vi "Load Save Config.vi"(8 "error in (no error)":errorcluster, 10 "OM  Location":T1, 11 "Actions":T2=enum."Load") -> (0 "error out":errorcluster)   [LabVIEW 2009]
uses:
  Data Access Objects/Metadata/Persistant DAO Actions.ctl
  Data Access Objects/Metadata/LBCB Location.ctl
  ConfigPathActions.ctl
  Data Access Objects/Metadata/LBCB Number.ctl
  <vilib>/Utility/config.llb/NI_LVConfig.lvlib
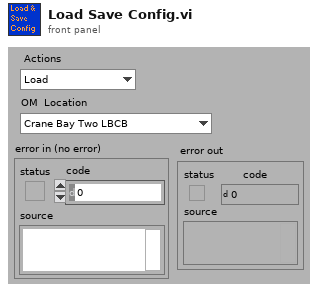
[diagram p1: front panel]
types:
  T1 = typedef "LBCB Location.ctl" = enum16{"Crane Bay Two LBCB", "Crane Bay One LBCB", "5th Scale Two LBCB", "5th Scale One LBCB", "Portable LBCB"}
  T2 = typedef "Persistant DAO Actions.ctl" = enum16{"Init", "Get", "Set", "Load", "Save"}
  T3 = typedef "ConfigPathActions.ctl" = enum16{"Init", "Application", "MixedMode", "ControlLoop", "Calibration", "System", "Change Location"}
  T4 = typedef "LBCB Number.ctl" = enum16{"LBCB1", "LBCB2"}
  T5 = typedef "NI_LVConfig.lvlib/Config Data RefNum.ctl" = refnum<k1>
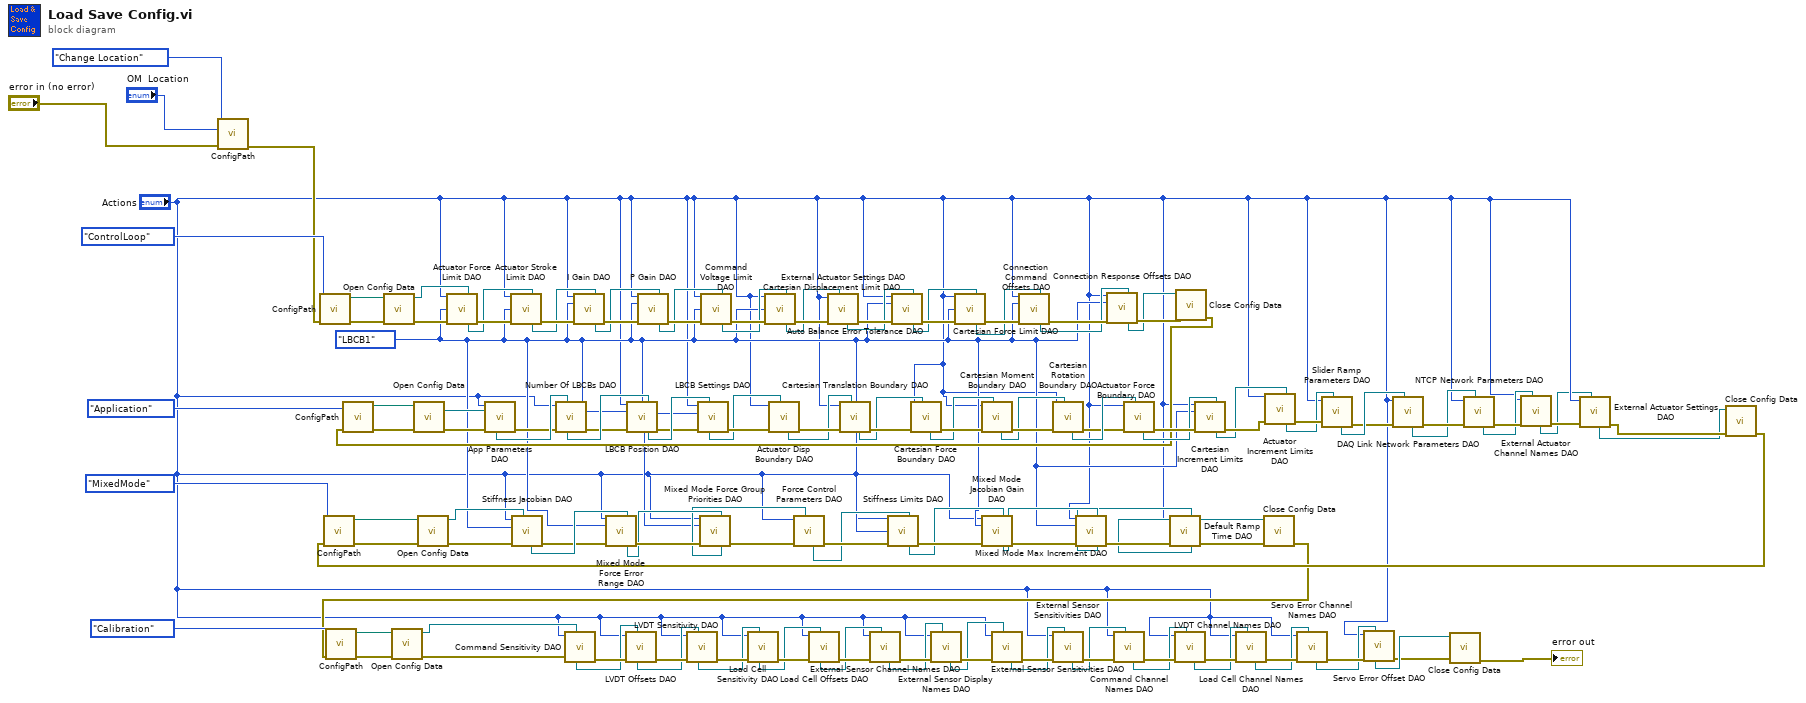
[diagram p0: block diagram]
diagram:
  w12 = LBCB_Number."LBCB1" ("LBCB Number")
  n1 = call "ConfigPath.vi"("error in (no error)"="error in (no error)", "OM  Location"="OM  Location", "Config Path Actions"=ConfigPathActions."Change Location") -> ("error out"=w89:errorcluster)  [unwired: 8 out]
  n2 = call "ConfigPath.vi"("error in (no error)"=w89, "Config Path Actions"=ConfigPathActions."ControlLoop") -> ("error out"=w130:errorcluster, "Path"=w129:path)  [unwired: 1 in, 7 out]
  n3 = call <vilib>:"Open Config Data.vi"("error in (no error)"=w130, "configuration file path"=w129) -> ("error out"=w127:errorcluster, "refnum"=w126:T5)  [unwired: 7 in, 1 out]
  n4 = call "Actuator Force Limit DAO.vi"("Actuator Force Limit Actions"="Actions", "Config Ref Number"=w126, "ID"=w12, "error in (no error)"=w127) -> ("Config Ref Number out"=w117:T5, "error out"=w125:errorcluster)  [unwired: 1 in, 9 out]
  n5 = call "Actuator Stroke Limit DAO.vi"("Actuator Stroke Limit Actions"="Actions", "Config Ref Number"=w117, "ID"=w12, "error in (no error)"=w125) -> ("Config Ref Number out"=w116:T5, "error out"=w124:errorcluster)  [unwired: 1 in, 9 out]
  n6 = call "I Gain DAO.vi"("I Gain Actions"="Actions", "Config Ref Number"=w116, "LBCB Number"=w12, "error in (no error)"=w124) -> ("Config Ref Number out"=w115:T5, "error out"=w123:errorcluster)  [unwired: 1 in, 9 out]
  n7 = call "P Gain DAO.vi"("P Gain Actions"="Actions", "Config Ref Number"=w115, "LBCB Number"=w12, "error in (no error)"=w123) -> ("Config Ref Number out"=w114:T5, "error out"=w122:errorcluster)  [unwired: 1 in, 9 out]
  n8 = call "Command Voltage Limit DAO.vi"("Actuator Stroke Limit Actions"="Actions", "Config Ref Number"=w114, "ID"=w12, "error in (no error)"=w122) -> ("Config Ref Number out"=w113:T5, "error out"=w121:errorcluster)  [unwired: 1 in, 9 out]
  n9 = call "Cartesian Displacement Limit DAO.vi"("Cartesian Displacement Limit Actions"="Actions", "Config Ref Number"=w113, "ID"=w12, "error in (no error)"=w121) -> ("Config Ref Number out"=w112:T5, "error out"=w120:errorcluster)  [unwired: 1 in, 9 out]
  n10 = call "External Actuator Settings DAO.vi"("refnum"=w112, "error in (no error)"=w120, "Persistent DAO Actions"="Actions") -> ("error out"=w119:errorcluster, "refnum out"=w111:T5)  [unwired: 2 in, 5 out]
  n11 = call "Auto Balance Error Tolerance DAO.vi"("Auto Balance Increment Actions"="Actions", "Config Ref"=w111, "LBCB Number"=w12, "error in (no error)"=w119) -> ("Config Ref  out"=w110:T5, "error out"=w118:errorcluster)  [unwired: 1 in, 9 out]
  n12 = call "Cartesian Force Limit DAO.vi"("Cartesian Force Limit Actions"="Actions", "Config Ref Number"=w110, "ID"=w12, "error in (no error)"=w118) -> ("Config Ref Number out"=w15:T5, "error out"=w19:errorcluster)  [unwired: 1 in, 9 out]
  n13 = call "Connection Command Offsets DAO.vi"("Actions"="Actions", "Config Ref Number"=w15, "LBCB Number"=w12, "error in (no error)"=w19) -> ("Config Ref Number out"=w14:T5, "error out"=w18:errorcluster)  [unwired: 9 in, 1 out]
  n14 = call "Connection Response Offsets DAO.vi"("Actions"="Actions", "Config Ref Number"=w14, "LBCB Number"=w12, "error in (no error)"=w18) -> ("Config Ref Number out"=w13:T5, "error out"=w17:errorcluster)  [unwired: 9 in, 1 out]
  n15 = call <vilib>:"Close Config Data.vi"("error in (no error)"=w17, "refnum"=w13) -> ("error out"=w16:errorcluster)  [unwired: 1 in, 8 out]
  n16 = call "ConfigPath.vi"("error in (no error)"=w16, "Config Path Actions"=ConfigPathActions."Application") -> ("error out"=w109:errorcluster, "Path"=w108:path)  [unwired: 1 in, 7 out]
  n17 = call <vilib>:"Open Config Data.vi"("error in (no error)"=w109, "configuration file path"=w108) -> ("error out"=w106:errorcluster, "refnum"=w105:T5)  [unwired: 7 in, 1 out]
  n18 = call "App Parameters DAO.vi"("config ref in"=w105, "error in (no error)"=w106, "Actions"="Actions") -> ("error out"=w87:errorcluster, "config ref out"=w88:T5)  [unwired: 1 in, 6 out]
  n19 = call "Number Of LBCBs DAO.vi"("Config ref in"=w88, "error in (no error)"=w87, "Actions"="Actions") -> ("error out"=w92:errorcluster, "Config ref out"=w94:T5)  [unwired: 2 in, 5 out]
  n20 = call "LBCB Position DAO.vi"("LBCB Settings Actions"="Actions", "Config Ref Number"=w94, "LBCB Number"=w12, "error in (no error)"=w92) -> ("Config Ref Number out"=w93:T5, "error out"=w91:errorcluster)  [unwired: 1 in, 9 out]
  n21 = call "LBCB Settings DAO.vi"("Config ref in"=w93, "error in (no error)"=w91, "LBCB Number"=w12, "Actions"="Actions") -> ("error out"=w81:errorcluster, "Config ref out"=w80:T5)  [unwired: 1 in, 5 out]
  n22 = call "Actuator Disp Boundary DAO.vi"("refnum in"=w80, "error in (no error)"=w81, "Actions"="Actions") -> ("error out"=w85:errorcluster, "refnum out"=w79:T5)  [unwired: 1 in, 6 out]
  n23 = call "Cartesian Translation Boundary DAO.vi"("refnum in"=w79, "error in (no error)"=w85, "Actions"="Actions") -> ("error out"=w84:errorcluster, "refnum out"=w78:T5)  [unwired: 1 in, 6 out]
  n24 = call "Cartesian Force Boundary DAO.vi"("refnum in"=w78, "error in (no error)"=w84, "Actions"="Actions") -> ("error out"=w83:errorcluster, "refnum out"=w77:T5)  [unwired: 1 in, 6 out]
  n25 = call "Cartesian Moment Boundary DAO.vi"("refnum in"=w77, "error in (no error)"=w83, "Actions"="Actions") -> ("error out"=w82:errorcluster, "refnum out"=w76:T5)  [unwired: 1 in, 6 out]
  n26 = call "Cartesian Rotation Boundary DAO.vi"("refnum in"=w76, "error in (no error)"=w82, "Actions"="Actions") -> ("error out"=w74:errorcluster, "refnum out"=w75:T5)  [unwired: 1 in, 6 out]
  n27 = call "Actuator Force Boundary DAO.vi"("refnum in"=w75, "error in (no error)"=w74, "Actions"="Actions") -> ("error out"=w21:errorcluster, "refnum out"=w20:T5)  [unwired: 1 in, 6 out]
  n28 = call "Cartesian Increment Limits DAO.vi"("Actions"="Actions", "Config Ref Number"=w20, "LBCB Number"=w12, "error in (no error)"=w21) -> ("Config Ref Number out"=w8:T5, "error out"=w11:errorcluster)  [unwired: 9 in, 1 out]
  n29 = call "Actuator Increment Limits DAO.vi"("Actions"="Actions", "Config Ref Number"=w8, "error in (no error)"=w11) -> ("Config Ref Number out"=w9:T5, "error out"=w10:errorcluster)  [unwired: 10 in, 1 out]
  n30 = call "Slider Ramp Parameters DAO.vi"("refnum in"=w9, "error in (no error)"=w10, "Persistent DAO Actions"="Actions") -> ("error out"=w67:errorcluster, "refnum out"=w68:T5)  [unwired: 1 in, 6 out]
  n31 = call "DAQ Link Network Parameters DAO.vi"("refnum"=w68, "error in (no error)"=w67, "Persistent DAO Actions"="Actions") -> ("error out"=w31:errorcluster, "refnum out"=w30:T5)  [unwired: 1 in, 6 out]
  n32 = call "NTCP Network Parameters DAO.vi"("refnum"=w30, "error in (no error)"=w31, "Persistent DAO Actions"="Actions") -> ("error out"=w7:errorcluster, "refnum out"=w4:T5)  [unwired: 6 in, 1 out]
  n33 = call "External Actuator Channel Names DAO.vi"("refnum"=w4, "error in (no error)"=w7, "Persistent DAO Actions"="Actions") -> ("error out"=w6:errorcluster, "refnum out"=w2:T5)  [unwired: 6 in, 1 out]
  n34 = call "External Actuator Settings DAO.vi"("refnum"=w2, "error in (no error)"=w6, "Persistent DAO Actions"="Actions") -> ("error out"=w5:errorcluster, "refnum out"=w1:T5)  [unwired: 6 in, 1 out]
  n35 = call <vilib>:"Close Config Data.vi"("error in (no error)"=w5, "refnum"=w1) -> ("error out"=w86:errorcluster)  [unwired: 1 in, 8 out]
  n36 = call "ConfigPath.vi"("error in (no error)"=w86, "Config Path Actions"=ConfigPathActions."MixedMode") -> ("error out"=w104:errorcluster, "Path"=w103:path)  [unwired: 1 in, 7 out]
  n37 = call <vilib>:"Open Config Data.vi"("error in (no error)"=w104, "configuration file path"=w103) -> ("error out"=w98:errorcluster, "refnum"=w101:T5)  [unwired: 7 in, 1 out]
  n38 = call "Stiffness Jacobian DAO.vi"("refnum in"=w101, "error in (no error)"=w98, "LBCB Number"=w12, "Actions"="Actions") -> ("error out"=w97:errorcluster, "refnum out"=w100:T5)  [unwired: 1 in, 5 out]
  n39 = call "Mixed Mode Force Error Range DAO.vi"("Force Error Range Actions"="Actions", "Config Ref Number"=w100, "LBCB Number"=w12, "error in (no error)"=w97) -> ("Config Ref Number out"=w28:T5, "error out"=w29:errorcluster)  [unwired: 1 in, 9 out]
  n40 = call "Mixed Mode Force Group Priorities DAO.vi"("Force Error Range Actions"="Actions", "Config Ref Number"=w28, "LBCB Number"=w12, "error in (no error)"=w29) -> ("Config Ref Number out"=w23:T5, "error out"=w27:errorcluster)  [unwired: 9 in, 1 out]
  n41 = call "Force Control Parameters DAO.vi"("Config Ref Number"=w23, "error in (no error)"=w27, "DAO Actions"="Actions") -> ("error out"=w26:errorcluster, "Config Ref Number out"=w24:T5)  [unwired: 6 in, 1 out]
  n42 = call "Stiffness Limits DAO.vi"("Cartesian Force Limit Actions"="Actions", "Config Ref Number"=w24, "ID"=w12, "error in (no error)"=w26) -> ("Config Ref Number out"=w22:T5, "error out"=w25:errorcluster)  [unwired: 9 in, 1 out]
  n43 = call "Mixed Mode Jacobian Gain DAO.vi"("Jacobian Gain Actions"="Actions", "Config Ref Number"=w22, "LBCB Number"=w12, "error in (no error)"=w25) -> ("Config Ref Number out"=w99:T5, "error out"=w96:errorcluster)  [unwired: 1 in, 9 out]
  n44 = call "Mixed Mode Max Increment DAO.vi"("Max Increment Actions"="Actions", "Config Ref Number"=w99, "LBCB Number"=w12, "error in (no error)"=w96) -> ("Config Ref Number out"=w33:T5, "error out"=w35:errorcluster)  [unwired: 1 in, 9 out]
  n45 = call "Default Ramp Time DAO.vi"("Ramp Time Actions"="Actions", "Config Ref Number"=w33, "error in (no error)"=w35) -> ("Config Ref Number out"=w32:T5, "error out"=w34:errorcluster)  [unwired: 1 in, 10 out]
  n46 = call <vilib>:"Close Config Data.vi"("error in (no error)"=w34, "refnum"=w32) -> ("error out"=w59:errorcluster)  [unwired: 1 in, 8 out]
  n47 = call "ConfigPath.vi"("error in (no error)"=w59, "Config Path Actions"=ConfigPathActions."Calibration") -> ("error out"=w73:errorcluster, "Path"=w72:path)  [unwired: 1 in, 7 out]
  n48 = call <vilib>:"Open Config Data.vi"("error in (no error)"=w73, "configuration file path"=w72) -> ("error out"=w51:errorcluster, "refnum"=w50:T5)  [unwired: 7 in, 1 out]
  n49 = call "Command Sensitivity DAO.vi"("Config Ref  In"=w50, "error in (no error)"=w51, "Actions"="Actions") -> ("error out"=w66:errorcluster, "Config Ref Out"=w58:T5)  [unwired: 2 in, 5 out]
  n50 = call "LVDT Offsets DAO.vi"("Config Ref  In"=w58, "error in (no error)"=w66, "Actions"="Actions") -> ("error out"=w65:errorcluster, "Config Ref Out"=w57:T5)  [unwired: 2 in, 5 out]
  n51 = call "LVDT Sensitivity DAO.vi"("Config Ref  In"=w57, "error in (no error)"=w65, "Actions"="Actions") -> ("error out"=w64:errorcluster, "Config Ref Out"=w56:T5)  [unwired: 2 in, 5 out]
  n52 = call "Load Cell Sensitivity DAO.vi"("Config Ref  In"=w56, "error in (no error)"=w64, "Actions"="Actions") -> ("error out"=w63:errorcluster, "Config Ref Out"=w55:T5)  [unwired: 2 in, 5 out]
  n53 = call "Load Cell Offsets DAO.vi"("Config Ref  In"=w55, "error in (no error)"=w63, "Actions"="Actions") -> ("error out"=w62:errorcluster, "Config Ref Out"=w54:T5)  [unwired: 2 in, 5 out]
  n54 = call "External Sensor Channel Names DAO.vi"("refnum"=w54, "error in (no error)"=w62, "Persistent DAO Actions"="Actions") -> ("error out"=w61:errorcluster, "refnum out"=w53:T5)  [unwired: 1 in, 6 out]
  n55 = call "External Sensor Display Names DAO.vi"("refnum"=w53, "error in (no error)"=w61, "Persistent DAO Actions"="Actions") -> ("error out"=w60:errorcluster, "refnum out"=w52:T5)  [unwired: 1 in, 6 out]
  n56 = call "External Sensor Sensitivities DAO.vi"("refnum"=w52, "error in (no error)"=w60, "Persistent DAO Actions"="Actions") -> ("error out"=w45:errorcluster, "refnum out"=w40:T5)  [unwired: 1 in, 6 out]
  n57 = call "External Sensor Sensitivities DAO.vi"("refnum"=w40, "error in (no error)"=w45, "Persistent DAO Actions"="Actions") -> ("error out"=w46:errorcluster, "refnum out"=w44:T5)  [unwired: 1 in, 6 out]
  n58 = call "Command Channel Names DAO.vi"("Config Ref  In"=w44, "error in (no error)"=w46, "Actions"="Actions") -> ("error out"=w47:errorcluster, "Config Ref Out"=w43:T5)  [unwired: 2 in, 5 out]
  n59 = call "LVDT Channel Names DAO.vi"("Config Ref  In"=w43, "error in (no error)"=w47, "Actions"="Actions") -> ("error out"=w48:errorcluster, "Config Ref Out"=w42:T5)  [unwired: 2 in, 5 out]
  n60 = call "Load Cell Channel Names DAO.vi"("Config Ref  In"=w42, "error in (no error)"=w48, "Actions"="Actions") -> ("error out"=w49:errorcluster, "Config Ref Out"=w41:T5)  [unwired: 2 in, 5 out]
  n61 = call "Servo Error Channel Names DAO.vi"("Config Ref  In"=w41, "error in (no error)"=w49, "Actions"="Actions") -> ("error out"=w39:errorcluster, "Config Ref Out"=w38:T5)  [unwired: 2 in, 5 out]
  n62 = call "Servo Error Offset DAO.vi"("Config Ref  In"=w38, "error in (no error)"=w39, "Actions"="Actions") -> ("error out"=w36:errorcluster, "Config Ref Out"=w37:T5)  [unwired: 2 in, 5 out]
  n63 = call <vilib>:"Close Config Data.vi"("error in (no error)"=w36, "refnum"=w37) -> ("error out"=→"error out":errorcluster)  [unwired: 1 in, 8 out]
